vi "Test GUI.vi"() -> ()   [LabVIEW 2021, in "TemplateGUIOpenGDSActiveObject.lvlib"]
uses:
  TemplateGUIOpenGDSActiveObject.lvlib
  TemplateGUI/TemplateGUI.lvclass
panel:
  in  "Stop":bool
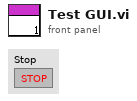
[diagram p1: front panel]
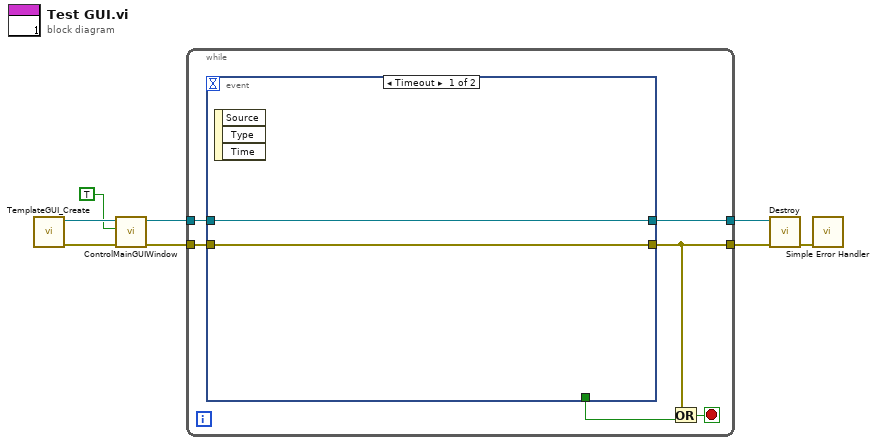
[diagram p0: block diagram]
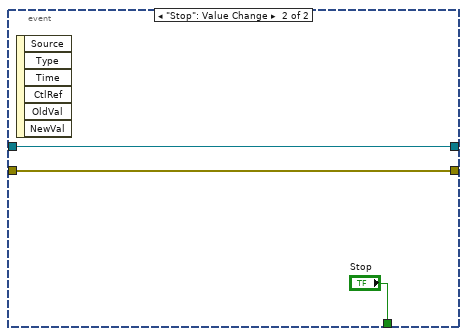
[diagram p2: hidden frame]
diagram:
  n1 = call "TemplateGUI_Create.vi"() -> ("ErrorOut"=w8:errorcluster, "ReferenceOut"=w4:refnum<class "TemplateGUI.lvclass">)  [unwired: 10 in]
  n2 = call "ControlMainGUIWindow.vi"("ErrorIn"=w8, "ShowProcessWindow"=TRUE, "ReferenceIn"=w4) -> ("ErrorOut"=w7:errorcluster, "ReferenceOut"=w2:refnum<class "TemplateGUI.lvclass">)  [unwired: 6 in, 1 out]
  n3 = while {
    tunnel: w7 -> [w14]
    tunnel: w2 -> [w12]
    tunnel: [w10] -> w1
    tunnel: [w13] -> w6
    stop <- w9 stop-if-true
    n4 = event shown="[0] Timeout" {
      selector: _ -> [_ _]
      dyn-events: _ -> [_ _]
      timeout: _ -> [_ _]
      tunnel: w14 -> [w16 w19]
      tunnel: w12 -> [w15 w17]
      tunnel: [_ "Stop"] -> w11
      tunnel: [w15 w17] -> w10
      tunnel: [w16 w19] -> w13
      event Timeout {
        n5 = event-data() -> ()  [unwired: 1 in, 3 out]
      }
      event "Stop": Value Change {
        n6 = event-data() -> ()  [unwired: 1 in, 6 out]
      }
    }
    n7 = Or(x=w13, y=w11) -> (x .or. y?=w9:bool)
  }
  n8 = call-dynamic "Destroy.vi"("ErrorIn"=w6, "ReferenceIn"=w1) -> ("ErrorOut"=w5:errorcluster)  [unwired: 8 in, 1 out]
  n9 = call <vilib>:"Simple Error Handler.vi"("error in (no error)"=w5) -> ()  [unwired: 4 in, 5 out]
